vi "strain_9215_v2.vi"() -> ()   [LabVIEW 2014]
uses:
  <vilib>/rvi/Emulation/niFpgaGetClockAttributes.vi
  <vilib>/rvi/Emulation/niFpgaSctlEmulationGetInTimedLoop.vi
  <vilib>/rvi/Emulation/niFpgaEmulationReportErrorSimple.vi
  <vilib>/rvi/Emulation/niFpgaProcessEmulError.vi
  <vilib>/rvi/interface/RandomDataEmulation/nirviRandomDataMultiElementFPGAFIFO.vi
  <instcachedir>/0/nirviRandomDataMultiElementFPGAFIFO_AD0CFC12EF974623A9C2E4184BC062B2.lvgen/nirviRandomDataMultiElementFPGAFIFO_AD0CFC12EF974623A9C2E4184BC062B2_025.vi
  <vilib>/rvi/interface/RandomDataEmulation/niFpgaRandomDataHandleErrors.vi
  <vilib>/rvi/Emulation/niFpgaCriticalErrorInLSC.vi
  <vilib>/rvi/eio/common/nirviEmuTemplateMethod_errors.vi
  <vilib>/rvi/DataTransferAndStorage/Container/XNode/niFpgaContainer.xnode
  <vilib>/rvi/interface/RandomDataEmulation/nirviRandomDataFpgaMultiElementTemplate.vi
  <vilib>/eio/EIONode/EIONode.xnode
  <vilib>/rvi/Analysis/measure/butterworth/XNode/niFpgaButterworthFilter.xnode
panel:
  in  "OP coeff.":fxp<+/-,20,8>
  in  "Count(mSec)":u32
  in  "Strain_p Avg2 coeff.":i32[](array[numeric])=[946630756, 63555534]
  in  "Strain_p Avg4 coeff.":i32[](array[numeric])=[946630756, 63555534]
  out "Strain_p (Avg2 w. f)":fxp<+/-,34,7>
  out "Strain_p (Avg4 w. f)":fxp<+/-,35,7>
  out "Strain_p (Avg2)":fxp<+/-,30,3>
  out "Strain_p (Avg4)":fxp<+/-,31,3>
  out "Strain_y (Avg2 w. f)":fxp<+/-,34,7>
  in  "Strain_y Avg2 coeff.":i32[](array[numeric])=[946630756, 63555534]
  out "Strain_y (Avg4 w. f)":fxp<+/-,35,7>
  in  "Strain_y Avg4 coeff.":i32[](array[numeric])=[946630756, 63555534]
  out "Strain_y (Avg2)":fxp<+/-,30,3>
  out "Strain_y (Avg4)":fxp<+/-,31,3>
  out "Fp_dc":fxp<+/-,32,10>
  out "Fy_dc":fxp<+/-,32,10>
  in  "Zero_y":bool
  in  "Zero_p":bool
  in  "S/F coeff_p":fxp<+/-,25,-10>
  in  "S/F coeff_y":fxp<+/-,25,-10>
  out "Force_p":fxp<+/-,32,10>
  in  "Strain selection_p":i16(ring) items=["Raw", "Avg.", "Avg. w. filter"]
  out "Strain_p (Avg8 w. f)":fxp<+/-,36,8>
  in  "Strain_p Avg8 coeff.":i32[](array[numeric])=[946630756, 63555534]
  out "Strain_p (Avg8)":fxp<+/-,36,4>
  out "Raw Strain_p":fxp<+/-,36,6>
  out "Mod6/AI3":fxp<+/-,36,4>
  in  "Strain gage reset_p":bool
  out "Strain_y (Avg8 w. f)":fxp<+/-,36,8>
  in  "Strain_y Avg8 coeff.":i32[](array[numeric])=[-898916953, 1957103773, 3888751]
  out "Strain_y (Avg8)":fxp<+/-,36,4>
  in  "Strain selection_y":i16(ring) items=["Raw", "Avg.", "Avg. w. filter"]
  in  "Ini coe.":bool
  out "Loop rate (kHz)":fxp<+/-,36,7>
  out "Force_y":fxp<+/-,32,10>
  out "Raw Strain_y":fxp<+/-,36,6>
  in  "Strain gage reset_y":bool
  out "Mod6/AI2":fxp<+/-,36,4>
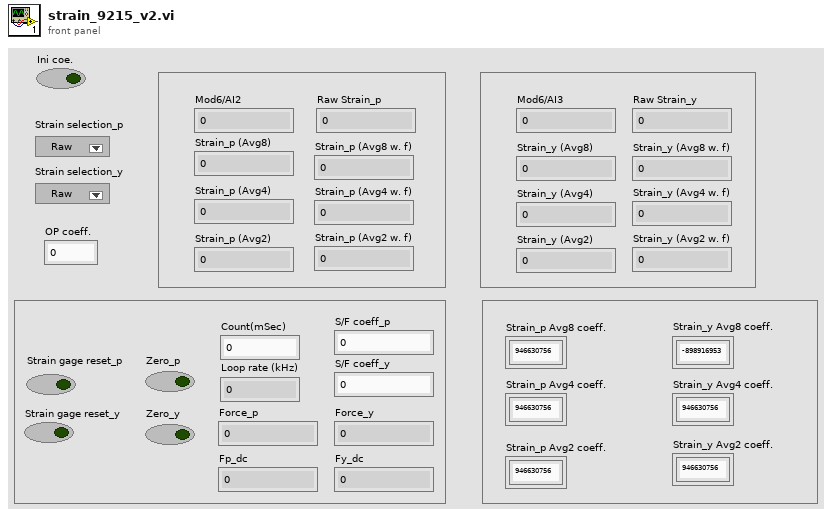
[diagram p1: front panel]
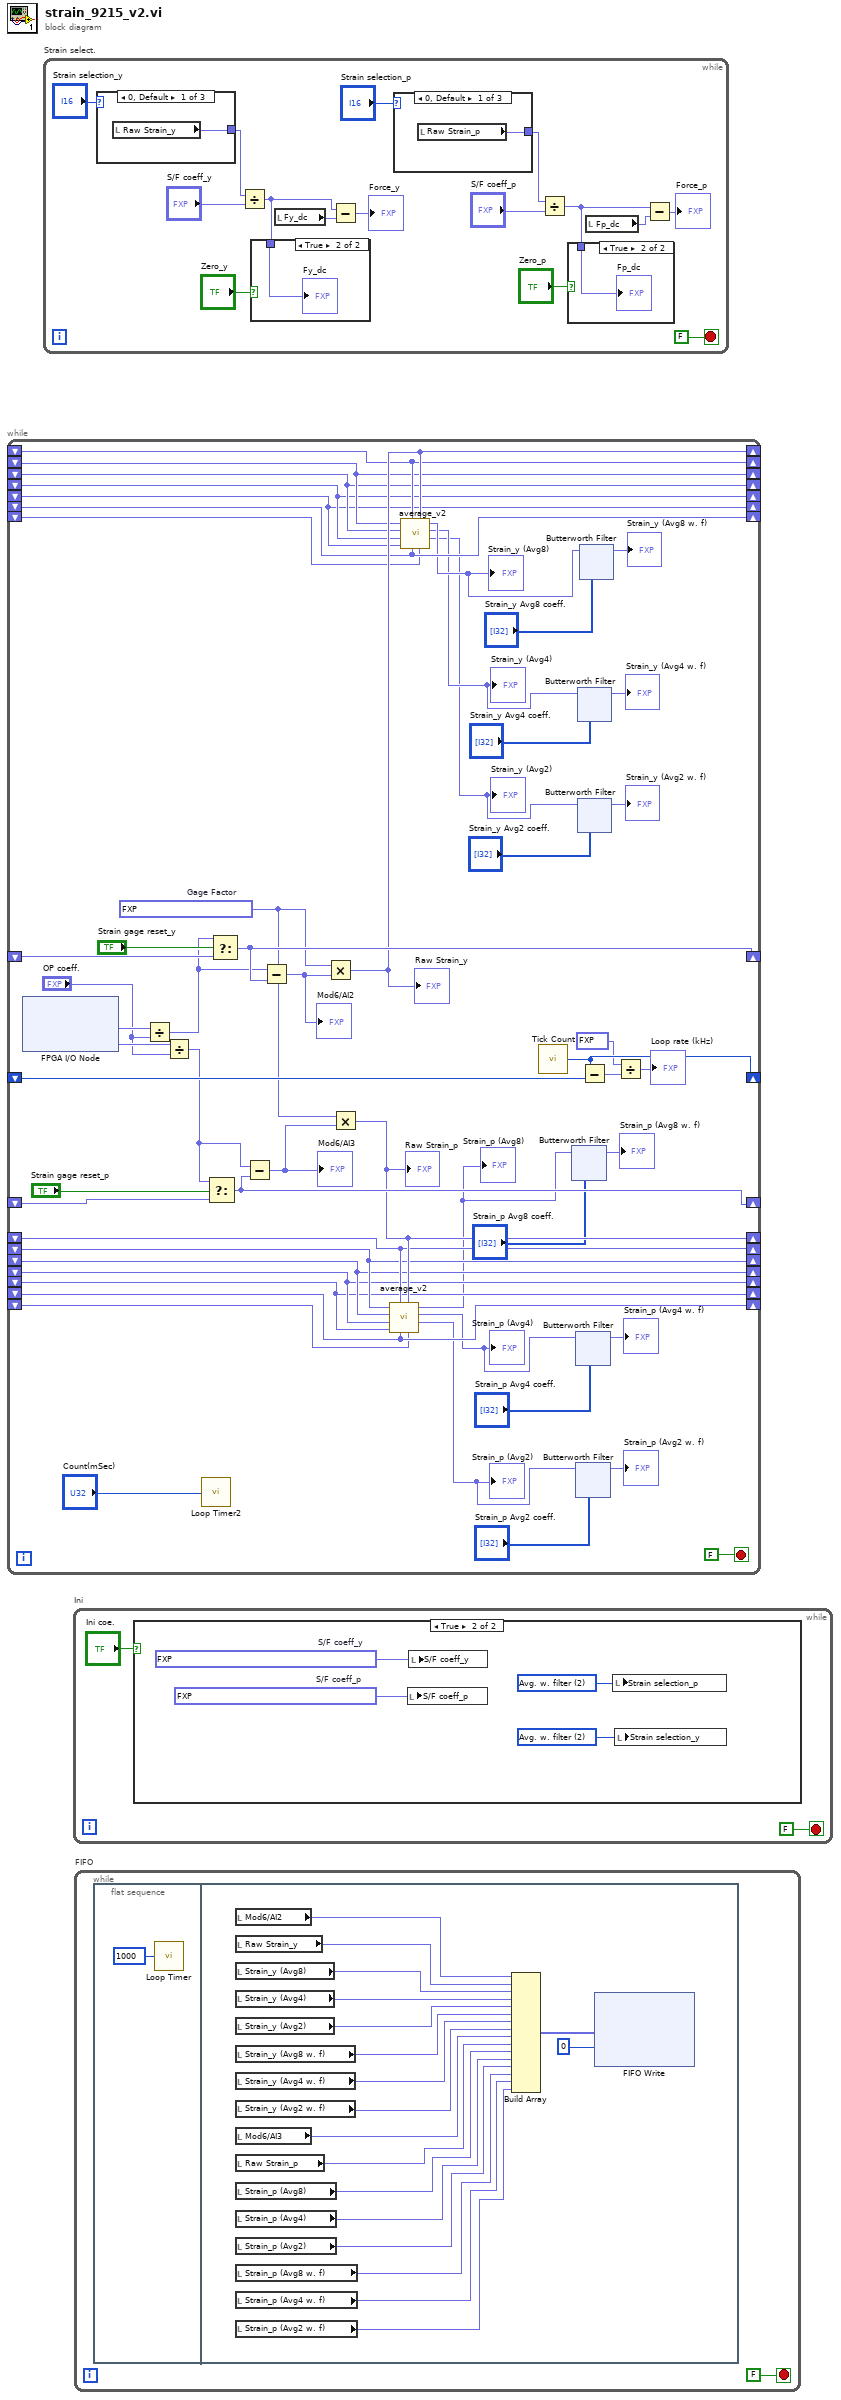
[diagram p0: block diagram]
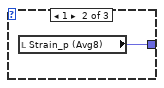
[diagram p4: hidden frame]
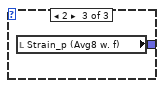
[diagram p5: hidden frame]
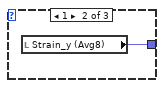
[diagram p6: hidden frame]
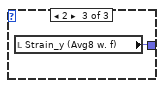
[diagram p7: hidden frame]
diagram:
  n1 = while {
    shift-right: [w54] -> _
    shift-left: _ -> [w55]
    shift-right: [w51] -> _
    shift-left: _ -> [w52]
    shift-right: [w46] -> _
    shift-left: _ -> [w45]
    shift-right: [w45] -> _
    shift-left: _ -> [w44]
    shift-right: [w44] -> _
    shift-left: _ -> [w43]
    shift-right: [w43] -> _
    shift-left: _ -> [w42]
    shift-right: [w42] -> _
    shift-left: _ -> [w41]
    shift-right: [w41] -> _
    shift-left: _ -> [w40]
    shift-right: [w40] -> _
    shift-left: _ -> [w39]
    shift-right: [w33] -> _
    shift-left: _ -> [w34]
    shift-right: [w30] -> _
    shift-left: _ -> [w29]
    shift-right: [w29] -> _
    shift-left: _ -> [w28]
    shift-right: [w28] -> _
    shift-left: _ -> [w27]
    shift-right: [w27] -> _
    shift-left: _ -> [w26]
    shift-right: [w26] -> _
    shift-left: _ -> [w25]
    shift-right: [w25] -> _
    shift-left: _ -> [w24]
    shift-right: [w24] -> _
    shift-left: _ -> [w23]
    stop <- FALSE stop-if-true
    w32 = fxp<+,20,2> 2.115001678466797  # Gage Factor
    n2 = xnode "FPGA I/O Node"() -> ("Mod3/AI1"=w5:fxp<+/-,20,5>, "Mod3/AI2"=w3:fxp<+/-,20,5>)  [unwired: 3 in, 3 out]
    n3 = Divide(x=w5, y="OP coeff.") -> (x/y=w4:fxp<+/-,41,18>)
    n4 = Divide(x=w3, y="OP coeff.") -> (x/y=w1:fxp<+/-,41,18>)
    n5 = call "Loop Timer2"("Count(mSec)"="Count(mSec)") -> ()  [unwired: 1 out]
    n6 = Select(t=w1, s="Strain gage reset_p", f=w34) -> (s? t:f=w33:fxp<+/-,41,18>)
    n7 = Select(t=w4, s="Strain gage reset_y", f=w55) -> (s? t:f=w54:fxp<+/-,41,18>)
    n8 = Subtract(x=w1, y=w33) -> (x-y=w31:fxp<+/-,30,-3>)
    "Mod6/AI3" <- w31
    n9 = Subtract(x=w4, y=w54) -> (x-y=w53:fxp<+/-,30,-3>)
    "Mod6/AI2" <- w53
    n10 = Multiply(x=w32, y=w53) -> (x*y=w46:fxp<+/-,41,6>)
    "Raw Strain_y" <- w46
    n11 = Multiply(x=w32, y=w31) -> (x*y=w30:fxp<+/-,50,-1>)
    "Raw Strain_p" <- w30
    n12 = call "average_v2.vi"("Numeric 8"=w23, "Numeric"=w30, "Numeric 7"=w24, "Numeric 2"=w29, "Numeric 6"=w25, "Numeric 5"=w26, "Numeric 4"=w27, "Numeric 3"=w28) -> ("Mean (2pt)"=w10:fxp<+/-,30,3>, "Mean (4pt)"=w12:fxp<+/-,31,3>, "Mean (8pt)"=w22:fxp<+/-,32,4>)  [unwired: 1 in]
    "Strain_p (Avg8)" <- w22
    "Strain_p (Avg4)" <- w12
    "Strain_p (Avg2)" <- w10
    n13 = call "average_v2.vi"("Numeric 8"=w39, "Numeric"=w46, "Numeric 7"=w40, "Numeric 2"=w45, "Numeric 6"=w41, "Numeric 5"=w42, "Numeric 4"=w43, "Numeric 3"=w44) -> ("Mean (2pt)"=w16:fxp<+/-,30,3>, "Mean (4pt)"=w19:fxp<+/-,31,3>, "Mean (8pt)"=w38:fxp<+/-,32,4>)  [unwired: 1 in]
    "Strain_y (Avg8)" <- w38
    "Strain_y (Avg4)" <- w19
    "Strain_y (Avg2)" <- w16
    n14 = call "Tick Count"() -> ("Tick Count(uSec)"=w51:u32)
    n15 = xnode "Butterworth Filter"("input data"=w22, "scaled coefficients"="Strain_p Avg8 coeff.") -> ("output data"=→"Strain_p (Avg8 w. f)":fxp<+/-,36,8>)  [unwired: 1 in]
    n16 = xnode "Butterworth Filter"("input data"=w12, "scaled coefficients"="Strain_p Avg4 coeff.") -> ("output data"=→"Strain_p (Avg4 w. f)":fxp<+/-,35,7>)  [unwired: 1 in]
    n17 = xnode "Butterworth Filter"("input data"=w10, "scaled coefficients"="Strain_p Avg2 coeff.") -> ("output data"=→"Strain_p (Avg2 w. f)":fxp<+/-,34,7>)  [unwired: 1 in]
    n18 = xnode "Butterworth Filter"("input data"=w19, "scaled coefficients"="Strain_y Avg4 coeff.") -> ("output data"=→"Strain_y (Avg4 w. f)":fxp<+/-,35,7>)  [unwired: 1 in]
    n19 = xnode "Butterworth Filter"("input data"=w16, "scaled coefficients"="Strain_y Avg2 coeff.") -> ("output data"=→"Strain_y (Avg2 w. f)":fxp<+/-,34,7>)  [unwired: 1 in]
    n20 = xnode "Butterworth Filter"("input data"=w38, "scaled coefficients"="Strain_y Avg8 coeff.") -> ("output data"=→"Strain_y (Avg8 w. f)":fxp<+/-,32,4>)  [unwired: 1 in]
    n21 = Subtract(x=w51, y=w52) -> (x-y=w49:fxp<+/-,32,16>)
    n22 = Divide(x=fxp<+,7,10> 1000.0, y=w49) -> (x/y=→"Loop rate (kHz)":fxp<+/-,40,27>)
  }
  n23 = while "Strain select." {
    stop <- FALSE stop-if-true
    n24 = case shown="0, Default" "Strain selection_y" {
      tunnel: [w124 w125 w126] -> w117
      frame 0, Default {
        n25 = local read "Raw Strain_y"() -> (w124:fxp<+/-,36,6>)
      }
      frame 1 {
        n26 = local read "Strain_y (Avg8)"() -> (w125:fxp<+/-,36,4>)
      }
      frame 2 {
        n27 = local read "Strain_y (Avg8 w. f)"() -> (w126:fxp<+/-,36,8>)
      }
    }
    n28 = Divide(x=w117, y="S/F coeff_y") -> (x/y=w110:fxp<+/-,32,10>)
    n29 = case shown="True" "Zero_y" {
      tunnel: w110 -> [_ w120]
      frame False {
      }
      frame True {
        "Fy_dc" <- w120
      }
    }
    n30 = local read "Fy_dc"() -> (w111:fxp<+/-,32,10>)
    n31 = Subtract(x=w110, y=w111) -> (x-y=→"Force_y":fxp<+/-,33,11>)
    n32 = case shown="0, Default" "Strain selection_p" {
      tunnel: [w121 w122 w123] -> w115
      frame 0, Default {
        n33 = local read "Raw Strain_p"() -> (w121:fxp<+/-,36,6>)
      }
      frame 1 {
        n34 = local read "Strain_p (Avg8)"() -> (w122:fxp<+/-,36,4>)
      }
      frame 2 {
        n35 = local read "Strain_p (Avg8 w. f)"() -> (w123:fxp<+/-,36,8>)
      }
    }
    n36 = Divide(x=w115, y="S/F coeff_p") -> (x/y=w107:fxp<+/-,32,10>)
    n37 = case shown="True" "Zero_p" {
      tunnel: w107 -> [_ w119]
      frame False {
      }
      frame True {
        "Fp_dc" <- w119
      }
    }
    n38 = local read "Fp_dc"() -> (w105:fxp<+/-,32,10>)
    n39 = Subtract(x=w107, y=w105) -> (x-y=→"Force_p":fxp<+/-,33,11>)
  }
  n40 = while "Ini" {
    stop <- FALSE stop-if-true
    n41 = case shown="True" "Ini coe." {
      frame False {
      }
      frame True {
        w129 = i16 2 items=["Raw", "Avg.", "Avg. w. filter"] ("Strain selection_p")
        w130 = i16 2 items=["Raw", "Avg.", "Avg. w. filter"] ("Strain selection_y")
        w132 = fxp<+/-,25,-10> -5.851034075021744e-07  # S/F coeff_p
        w131 = fxp<+/-,25,-10> -1.0477961041033268e-06  # S/F coeff_y
        n42 = local write "S/F coeff_p"(w132) -> ()
        n43 = local write "S/F coeff_y"(w131) -> ()
        n44 = local write "Strain selection_p"(w129) -> ()
        n45 = local write "Strain selection_y"(w130) -> ()
      }
    }
  }
  n46 = while "FIFO" {
    stop <- FALSE stop-if-true
    n47 = flat-sequence {
      frame #0 {
        n48 = call "Loop Timer"("Count(uSec)"=u32 1000) -> ()  [unwired: 1 out]
      }
      frame #1 {
        n49 = local read "Mod6/AI2"() -> (w152:fxp<+/-,36,4>)
        n50 = local read "Raw Strain_y"() -> (w151:fxp<+/-,36,6>)
        n51 = local read "Strain_y (Avg8)"() -> (w150:fxp<+/-,36,4>)
        n52 = local read "Strain_y (Avg4)"() -> (w149:fxp<+/-,31,3>)
        n53 = local read "Strain_y (Avg2)"() -> (w145:fxp<+/-,30,3>)
        n54 = local read "Strain_y (Avg8 w. f)"() -> (w146:fxp<+/-,36,8>)
        n55 = local read "Strain_y (Avg4 w. f)"() -> (w147:fxp<+/-,35,7>)
        n56 = local read "Strain_y (Avg2 w. f)"() -> (w136:fxp<+/-,34,7>)
        n57 = local read "Mod6/AI3"() -> (w144:fxp<+/-,36,4>)
        n58 = local read "Raw Strain_p"() -> (w143:fxp<+/-,36,6>)
        n59 = local read "Strain_p (Avg8)"() -> (w142:fxp<+/-,36,4>)
        n60 = local read "Strain_p (Avg4)"() -> (w141:fxp<+/-,31,3>)
        n61 = local read "Strain_p (Avg2)"() -> (w140:fxp<+/-,30,3>)
        n62 = local read "Strain_p (Avg8 w. f)"() -> (w139:fxp<+/-,36,8>)
        n63 = local read "Strain_p (Avg4 w. f)"() -> (w138:fxp<+/-,35,7>)
        n64 = local read "Strain_p (Avg2 w. f)"() -> (w135:fxp<+/-,34,7>)
        n65 = Build Array(w152, w151, w150, w149, w145, w146, w147, w136, w144, w143, w142, w141, w140, w139, w138, w135) -> (w137:fxp<+/-,40,8>[])
        n66 = xnode ("FIFO Write")("Element"=w137, "Timeout"=0) -> ()  [unwired: 1 in, 2 out]
      }
    }
  }
